vi "Loop.vi"(11 "Queue Actor in":refnum<class "Queue Actor.lvclass">) -> (3 "Queue Actor out":refnum<class "Queue Actor.lvclass">)   [LabVIEW 2021, in "Queue Actor.lvclass"]
uses:
  Queue Actor.lvclass
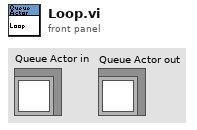
[diagram p1: front panel]
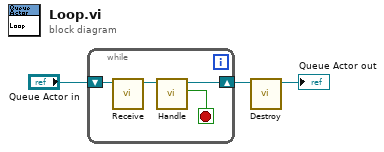
[diagram p0: block diagram]
diagram:
  n1 = while {
    shift-right: [w7] -> w2
    shift-left: "Queue Actor in" -> [w5]
    stop <- w6 stop-if-true
    n2 = call-dynamic "Receive.vi"("Queue Actor in"=w5) -> ("Queue Actor out"=w4:refnum<class "Queue Actor.lvclass">)  [unwired: 10 in]
    n3 = call-dynamic "Handle.vi"("Queue Actor in"=w4) -> ("Destroy?"=w6:bool, "Queue Actor out"=w7:refnum<class "Queue Actor.lvclass">)  [unwired: 9 in]
  }
  n4 = call-dynamic "Destroy.vi"("Queue Actor in"=w2) -> ("Queue Actor out"=→"Queue Actor out":refnum<class "Queue Actor.lvclass">)  [unwired: 10 in]
